vi "NT Logging Enable.vi"(11 "Enable":bool) -> ()   [LabVIEW 2025]
doc: "This is used to enable and disable the NT WPILogging feature where all NT writes are added to a log file to aid in debugging and tuning your robot."
uses:
  ntcoreffi.dll
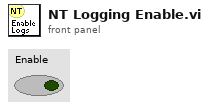
[diagram p1: front panel]
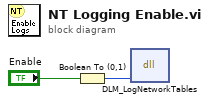
[diagram p0: block diagram]
diagram:
  n1 = Boolean To (0,1)(Boolean="Enable") -> (0, 1=w2:i16)
  n2 = dll-call lib="ntcoreffi.*" fn="DLM_LogNetworkTables"("enable"=w2) -> ()  [unwired: 5 in, 2 out]
